vi "Set DDS Amplitude Mv.vi"(8 "error in (no error)":errorcluster, 10 "amplitdude":i32, 11 "channel_index":u8) -> (0 "error out":errorcluster)   [LabVIEW 2021, in "vmmsolib.lvlib"]
doc: "DLL_API void WINAPI SetDDSAmplitudeMv(unsigned char channel_index, int amplitdude);"
uses:
  vmmsolib.lvlib
  vmmso.dll
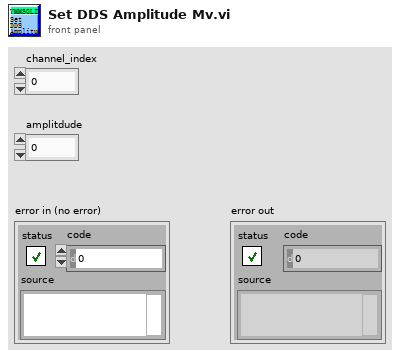
[diagram p1: front panel]
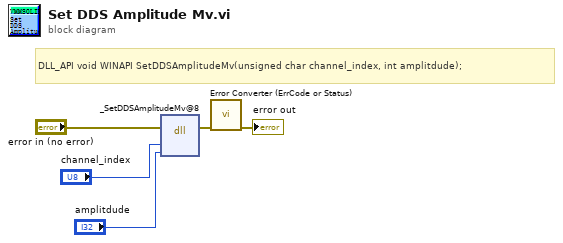
[diagram p0: block diagram]
diagram:
  # "DLL_API void WINAPI SetDDSAmplitudeMv(unsigned char channel_index, int amplitdude);"
  n1 = dll-call lib="D:/VmMsoSDK/demo-Labview/2021/vmmsolib/vmmso.*" fn="_SetDDSAmplitudeMv@8"(error in="error in (no error)", "channel_index"="channel_index", "amplitdude"="amplitdude") -> (error out=w2:errorcluster)  [unwired: 5 in, 1 out]
  n2 = call "Error Converter (ErrCode or Status).vi"("error in (no error)"=w2) -> ("error out"=→"error out":errorcluster)  [unwired: 10 in]
